vi "z_axis_ss_control_sin_est.vi"(5 "NS":u8=9, 7 "Ns+Nsd":i16, 8 "Ki_z":sgl, 9 "r":fxp<+/-,32,5>, 10 "u(k-1)":sgl format="%#_13g", 11 "Y(k): x":fxp<+/-,32,5>) -> (0 "sinusoid_est":fxp<+/-,32,5>, 3 "u_k (saturated)":fxp<+/-,32,5>)   [LabVIEW 2017]
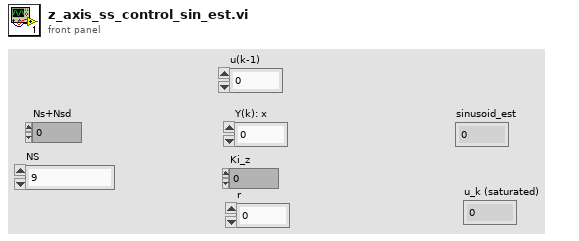
[diagram p1: front panel]
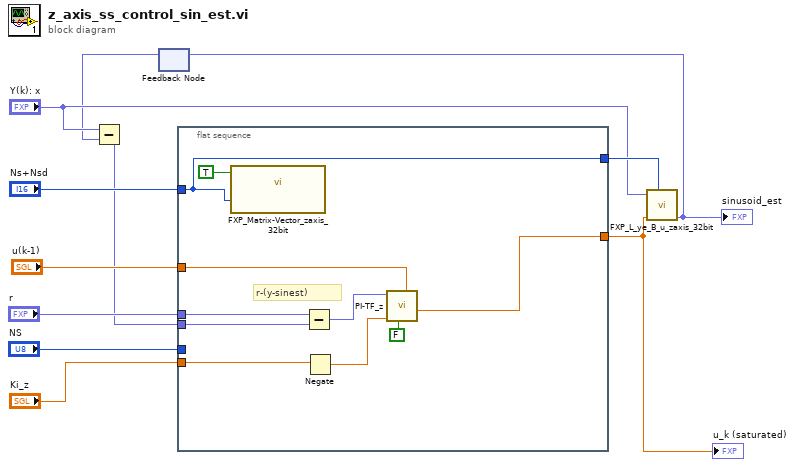
[diagram p0: block diagram]
diagram:
  n1 = feedback #1() -> (w2:fxp<+/-,32,5>)  [unwired: 1 in]
  n2 = Subtract(x="Y(k): x", y=w2) -> (x-y=w1:fxp<+/-,33,6>)
  n3 = flat-sequence {
    tunnel: "Ns+Nsd" -> [w21]
    tunnel: [w21] -> w9
    tunnel: [w15] -> w10
    tunnel: "NS" -> [_]
    tunnel: "r" -> [w16]
    tunnel: "Ki_z" -> [w14]
    tunnel: "u(k-1)" -> [w13]
    tunnel: w1 -> [w12]
    frame #0 {
      # "r-(y-sinest)"
      n4 = call "FXP_Matrix-Vector_zaxis_32bit.vi"("Ns_nsw"=w21, "inputValid"=TRUE) -> ()  [unwired: 9 in, 1 out]
      n5 = Subtract(x=w16, y=w12) -> (x-y=w18:fxp<+/-,34,7>)
      n6 = Negate(x=w14) -> (-x=w17:sgl)
      n7 = call "PI-TF_z.vi"("u(k-1)"=w13, "reset"=FALSE, "Ki"=w17, "e(k)"=w18) -> ("u(k)"=w15:sgl)  [unwired: 7 in]
    }
  }
  n8 = call "FXP_L_ye_B_u_zaxis_32bit.vi"("NS"=w9, "U(k): ux"=w10, "Y(k): x"="Y(k): x") -> ("sinusoid_est"=w4:fxp<+/-,32,5>)  [unwired: 7 in, 1 out]
  "sinusoid_est" <- w4
  n9 = feedback-in #1(w4) -> ()
  "u_k (saturated)" <- w10
